vi "Approximate Polygon (N-Side).vi"(5 "Epsilon % (Default: -1 ignore)":dbl=-1.0 format="%#_13g", 7 "Ensure Convex? (Default: True)":bool=TRUE, 8 "error in (no error)":errorcluster, 10 "N-Sides":u8, 11 "Points in":T1[](array[typedef])) -> (0 "error out":errorcluster, 3 "Points out":T1[](array[typedef]))   [LabVIEW 2020, in "shape.lvlib"]
doc: "Approximates a polygon with a convex hull so that the difference between the contour area of the original contour and the new polygon is minimal.\n\nIt uses a greedy algorithm for contracting two vertices into one in such a way that the additional area is minimal. Straight lines formed by each edge of the convex contour are drawn and the areas of the resulting triangles are considered. Each vertex will lie either on the original contour or outside it."
uses:
  shape.lvlib
  common/Image Point (Integer).ctl
  common/common.lvlib
  common/bin/gartoolkit_32-1.dll
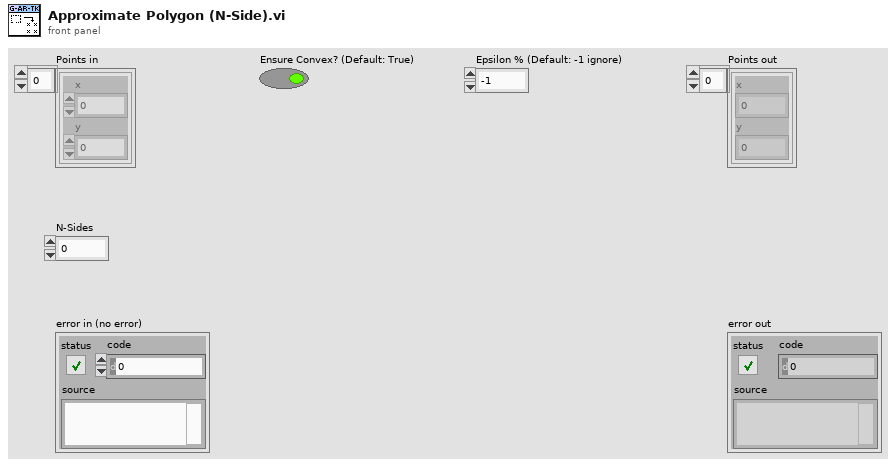
[diagram p1: front panel]
types:
  T1 = typedef "common.lvlib/Image Point (Integer).ctl" = cluster{"x":i32, "y":i32}
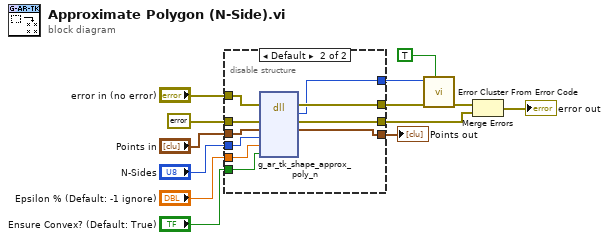
[diagram p0: block diagram]
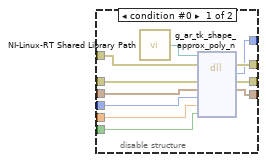
[diagram p2: hidden frame]
diagram:
  n1 = disable-structure shown="Default" {
    disable-tunnel: "error in (no error)" -> [w24 w34]
    disable-tunnel: errorcluster {"status"=FALSE, "code"=0, "source"=""} ("error constant") -> [w21 w33]
    disable-tunnel: "Points in" -> [w20 w32]
    disable-tunnel: "Epsilon % (Default: -1 ignore)" -> [w18 w31]
    disable-tunnel: "Ensure Convex? (Default: True)" -> [w17 w30]
    disable-tunnel: [w23 w29] -> w6
    disable-tunnel: [w22 w28] -> w5
    disable-tunnel: [w15 w27] -> w4
    disable-tunnel: [w16 w26] -> w3
    disable-tunnel: "N-Sides" -> [w19 w25]
    frame condition #0 {
      n2 = call "NI-Linux-RT Shared Library Path.vi"() -> ("Path"=w14:path)
      n3 = dll-call lib="?" fn="g_ar_tk_shape_approx_poly_n" ("g_ar_toolkit.*.*:g_ar_tk_image_draw_line")(path in=w14, error in=w24, "error_cluster"=w21, "points"=w20, "n_sides"=w19, "epsilon_pct"=w18, "ensure_convex"=w17) -> (error out=w23:errorcluster, w22:i32, "error_cluster"=w15:errorcluster, "points"=w16:T1[])  [unwired: 4 in, 1 out]
    }
    frame condition #1 (active) {
      n4 = dll-call lib="C:/serenial/lib/g-augmented-reality-toolkit/LabVIEW/common/bin/gartoolkit_*-1.*" fn="g_ar_tk_shape_approx_poly_n" ("g_ar_toolkit.*.*:g_ar_tk_image_draw_line")(error in=w34, "error_cluster"=w33, "points"=w32, "n_sides"=w25, "epsilon_pct"=w31, "ensure_convex"=w30) -> (error out=w29:errorcluster, w28:i32, "error_cluster"=w27:errorcluster, "points"=w26:T1[])  [unwired: 5 in, 1 out]
    }
  }
  "Points out" <- w3
  n5 = call <vilib>:"Error Cluster From Error Code.vi"("show call chain? (False)"=TRUE, "error in (no error)"=w6, "error code (0)"=w5) -> ("error out"=w12:errorcluster)  [unwired: 6 in]
  n6 = Merge Errors(w12, w4) -> (→"error out":errorcluster)
